vi "Analyze Data.vi"(8 "error in":errorcluster, 11 "cPAS in":refnum<class "cPAS.lvclass">) -> (0 "error out":errorcluster, 3 "cPAS out":refnum<class "cPAS.lvclass">)   [LabVIEW 2015, in "cPAS.lvclass"]
uses:
  cPAS.lvclass
  Reusable/PAS/Main/Read Cells.vi
  Reusable/PAS/Main/Read Data.vi
  Reusable/PAS/Main/Get Speaker State.vi
  Reusable/PAS/Data/Cell/Write derived.vi
  Reusable/PAS/Data/Cell/Read f0.vi
  Reusable/PAS/Cell/PAS Cell.lvclass
  Reusable/PAS/Data/Main/PAS Data.lvclass
  Reusable/PAS/Main/PAS.lvclass
  Reusable/PAS/Data/Cell/PAS Cell Data.lvclass
  Reusable/Instrument/Instrument.lvclass
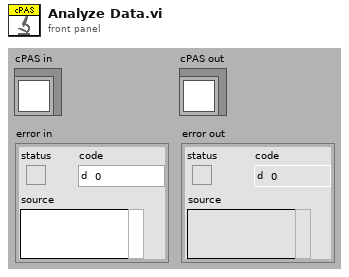
[diagram p1: front panel]
types:
  T1 = cluster{"f0":sgl, "IA":sgl, "Q":sgl, "max":dbl[], "deltaPhi":dbl, "tau":dbl, "noiseLim":dbl, "ext":dbl}
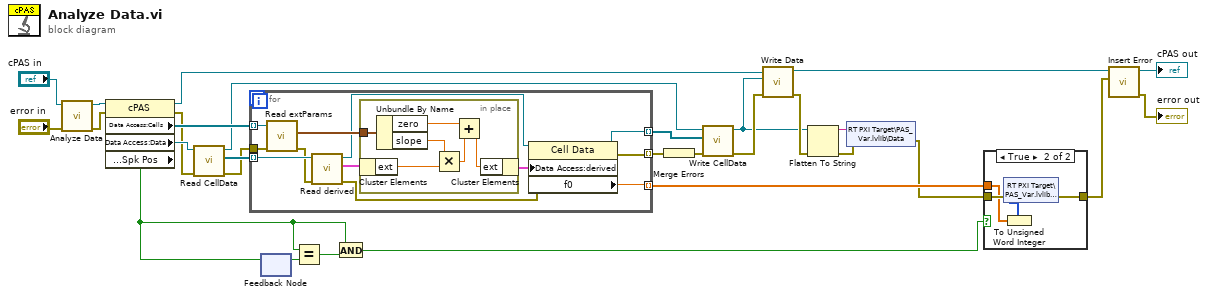
[diagram p0: block diagram]
diagram:
  n1 = call-parent "Analyze Data.vi"("error in"="error in", "PAS in"="cPAS in") -> ("error out"=w26:errorcluster, "PAS out"=w27:refnum<class "cPAS.lvclass">)  [unwired: 8 in]
  n2 = property class="cPAS"(reference=w27, error in=w26) -> (reference out=w18:refnum<class "cPAS.lvclass">, error out=w22:errorcluster, "Data Access:Cells"=w25:refnum<class "PAS Cell.lvclass">[], "Data Access:Data"=w23:refnum<class "PAS Data.lvclass">, "Data Access:Spk Pos"=w2:bool)
  n3 = call "Read CellData.vi"("error in"=w22, "PAS Data in"=w23) -> ("error out"=w21:errorcluster, "CellData"=w24:refnum<class "PAS Cell Data.lvclass">[], "PAS Data out"=w19:refnum<class "PAS Data.lvclass">)  [unwired: 7 in]
  n4 = for {
    tunnel: w25 -> [w41] mode=indexing
    tunnel: w24 -> [w40] mode=indexing
    tunnel: w21 -> [w37]
    tunnel: [w30] -> w16 mode=indexing
    tunnel: [w34] -> w20 mode=indexing
    tunnel: [w31] -> w7 mode=indexing
    n5 = call "Read extParams.vi"("error in"=w37, "PAS Cell in"=w41) -> ("error out"=w36:errorcluster, "extParams"=w38:cluster{"slope":sgl, "zero":sgl})  [unwired: 7 in, 1 out]
    n6 = call "Read derived.vi"("error in"=w36, "PAS Cell Data in"=w40) -> ("error out"=w33:errorcluster, "derived"=w39:T1, "PAS Cell Data out"=w35:refnum<class "PAS Cell Data.lvclass">)  [unwired: 7 in]
    n7 = in-place {
      in-place-border: w38 -> [w47]
      n8 = in-place-cluster #1(w39) -> ("ext"=w46:dbl)
      n9 = Unbundle By Name(w47) -> ("zero"=w43:sgl, "slope"=w42:sgl)
      n10 = Multiply(x=w42, y=w46) -> (x*y=w45:dbl)
      n11 = Add(x=w43, y=w45) -> (x+y=w44:dbl)
      n12 = in-place-cluster #1("ext"=w44) -> (w32:T1)
    }
    n13 = property class="Cell Data"(reference=w35, error in=w33, "Data Access:derived"=w32) -> (reference out=w34:refnum<class "PAS Cell Data.lvclass">, error out=w30:errorcluster, "f0"=w31:sgl)
  }
  n14 = feedback-in #2(w2) -> ()
  n15 = feedback #2() -> (w4:bool)  [unwired: 1 in]
  n16 = Equal?(x=w2, y=w4) -> (x = y?=w3:bool)
  n17 = And(x=w2, y=w3) -> (x .and. y?=w1:bool)
  n18 = Merge Errors(w16) -> (w15:errorcluster)
  n19 = call "Write CellData.vi"("error in"=w15, "CellData"=w20, "PAS Data in"=w19) -> ("error out"=w17:errorcluster, "PAS Data out"=w11:refnum<class "PAS Data.lvclass">)  [unwired: 7 in]
  n20 = call "Write Data.vi"("error in"=w17, "PAS Data.lvclass"=w11, "PAS in"=w18) -> ("error out"=w12:errorcluster, "PAS out"=w10:refnum<class "cPAS.lvclass">)  [unwired: 7 in]
  n21 = Flatten To String(anything=w11, error in (no error)=w12) -> (data string=w14:string, error out=w13:errorcluster)  [unwired: 2 in, 1 out]
  n22 = shared-variable "RT PXI Target\\PAS_Var.lvlib\\Data"(w14, error in=w13) -> (error out=w6:errorcluster)
  n23 = case shown="True" w1 {
    tunnel: w7 -> [_ w50]
    tunnel: w6 -> [w48 w52]
    tunnel: [w48 w51] -> w5
    frame False {
    }
    frame True {
      n24 = To Unsigned Word Integer(number=w50) -> (unsigned 16bit integer=w49:u16[])
      n25 = shared-variable "RT PXI Target\\PAS_Var.lvlib\\f0"(w49, error in=w52) -> (error out=w51:errorcluster)
    }
  }
  n26 = call "Insert Error.vi"("err"=w5, "Instrument in"=w10) -> ("error out"=→"error out":errorcluster, "Instrument out"=→"cPAS out":refnum<class "cPAS.lvclass">)  [unwired: 7 in, 1 out]
